vi "CTE_Analysis_Suite_InputMaker.vi"(11 "File Save Path":path=path "C:/TestInputMaker") -> ()   [LabVIEW 2012]
panel:
  in  "Crystal Symmetry":string(combo)="Monoclinic"
  out "Ready":bool=TRUE
  in  "New Phase":bool
  in  "Submit":bool
  in  "stop":bool
  in  "Clear All Fields":bool
  out "Saved As:":string="-25.csv"
  out "Submitted?":bool
  in  "hkl's and d-spacings (Å)":refnum<k7>(container) caption="hkl's and d-spacings (A)"
  in  "Error gamma":dbl
  in  "Error beta":dbl
  in  "Error alpha":dbl
  in  "Error c":dbl
  in  "Error b":dbl
  in  "Error a":dbl
  in  "Temp (°C)":dbl=25.0
  in  "gamma":dbl
  in  "beta":dbl
  in  "alpha":dbl
  in  "c":dbl
  in  "b":dbl
  in  "a":dbl
  in  "Chemical Formula or File Name (no subscripts)":string="FileName1"
  in  "Phase Name":string="NewPhase1"
  # "CTEAS InputMaker v0.2"
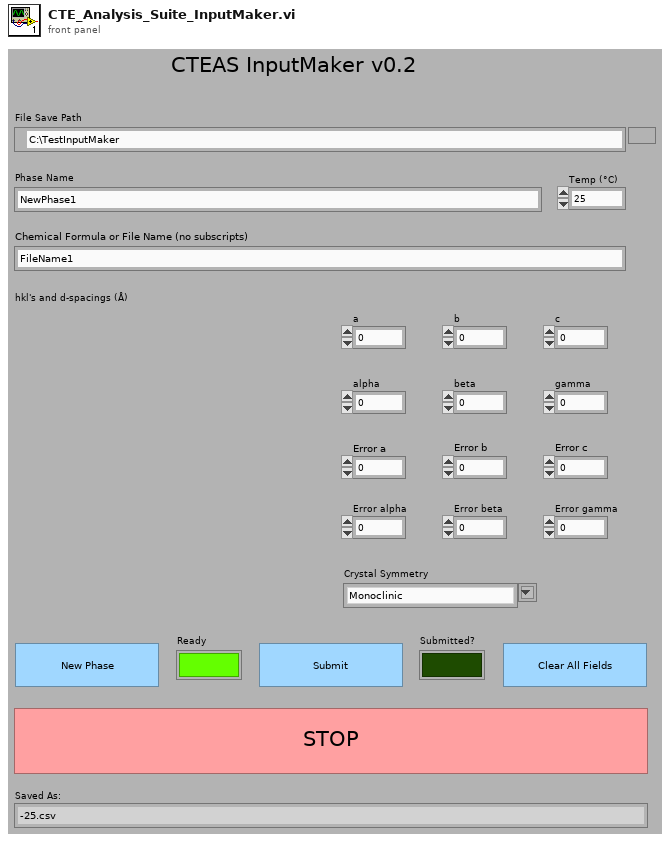
[diagram p1: front panel]
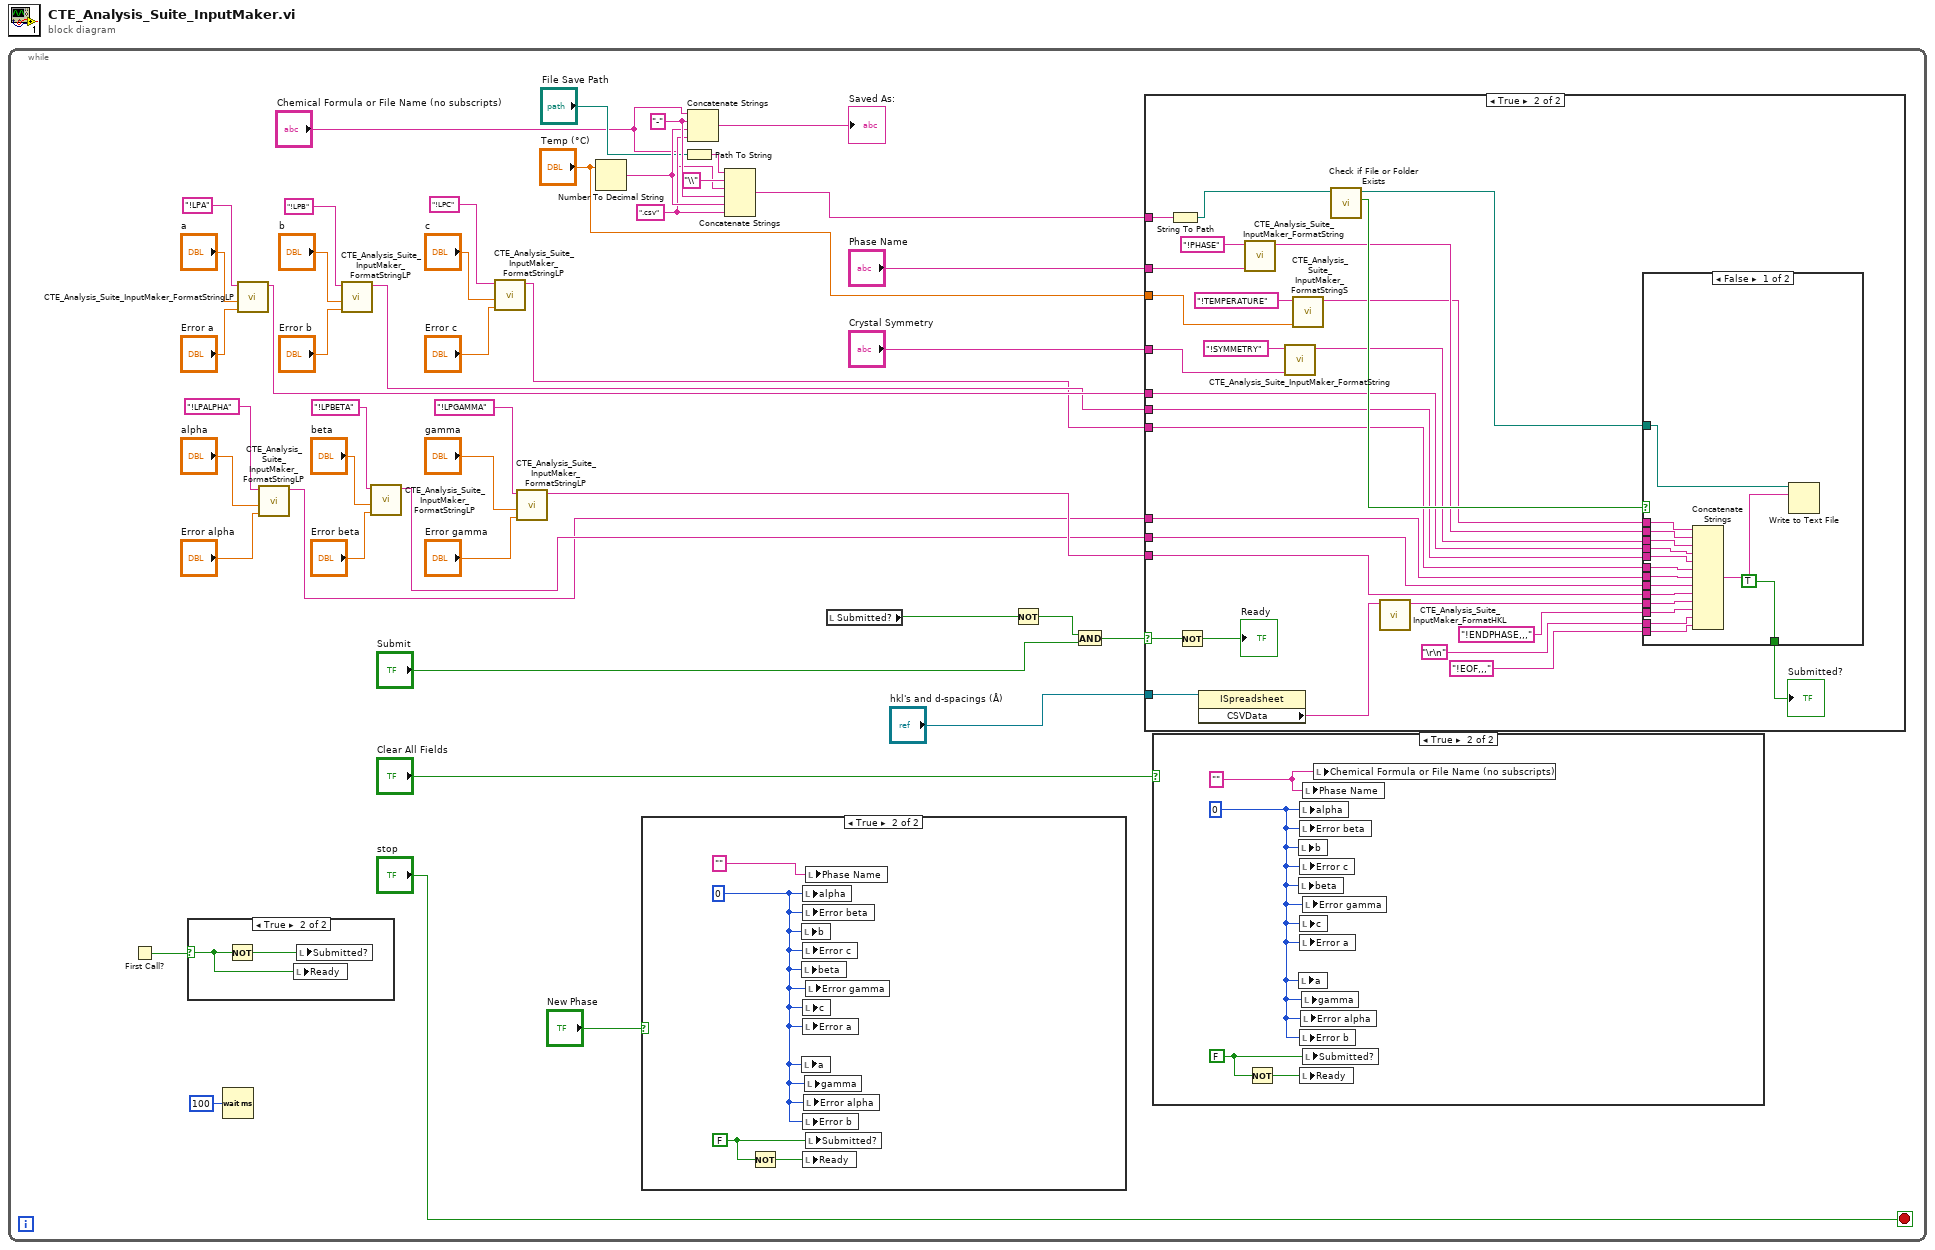
[diagram p0: block diagram]
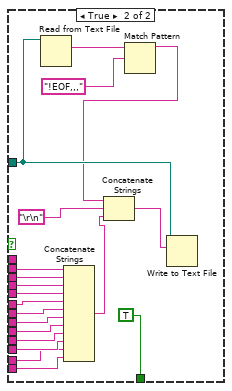
[diagram p6: hidden frame]
diagram:
  n1 = while {
    stop <- "stop" stop-if-true
    w41 = ".csv" ("string")
    w43 = "-" ("string")
    n2 = First Call?() -> (First Call?: T/F=w30:bool)
    n3 = case shown="True" w30 {
      selector: w30 -> [_ w51]
      frame False {
      }
      frame True {
        n4 = Not(x=w51) -> (.not. x?=w52:bool)
        n5 = local write "Ready"(w51) -> ()
        n6 = local write "Submitted?"(w52) -> ()
      }
    }
    n7 = Wait (ms)(milliseconds to wait=u32 100) -> ()  [unwired: 1 out]
    n8 = call "CTE_Analysis_Suite_InputMaker_FormatStringLP.vi"("ERROR"="Error a", "VALUE"="a", "NAME"="!LPA") -> ("Output"=w9:string)  [unwired: 8 in]
    n9 = call "CTE_Analysis_Suite_InputMaker_FormatStringLP.vi"("ERROR"="Error alpha", "VALUE"="alpha", "NAME"="!LPALPHA") -> ("Output"=w4:string)  [unwired: 8 in]
    n10 = call "CTE_Analysis_Suite_InputMaker_FormatStringLP.vi"("ERROR"="Error b", "VALUE"="b", "NAME"="!LPB") -> ("Output"=w8:string)  [unwired: 8 in]
    n11 = call "CTE_Analysis_Suite_InputMaker_FormatStringLP.vi"("ERROR"="Error beta", "VALUE"="beta", "NAME"="!LPBETA") -> ("Output"=w5:string)  [unwired: 8 in]
    n12 = call "CTE_Analysis_Suite_InputMaker_FormatStringLP.vi"("ERROR"="Error c", "VALUE"="c", "NAME"="!LPC") -> ("Output"=w7:string)  [unwired: 8 in]
    n13 = call "CTE_Analysis_Suite_InputMaker_FormatStringLP.vi"("ERROR"="Error gamma", "VALUE"="gamma", "NAME"="!LPGAMMA") -> ("Output"=w6:string)  [unwired: 8 in]
    n14 = Number To Decimal String(number="Temp (°C)") -> (decimal integer string=w42:string)  [unwired: 1 in]
    n15 = case shown="True" "New Phase" {
      frame False {
      }
      frame True {
        w50 = FALSE
        w48 = 0
        n16 = Not(x=w50) -> (.not. x?=w49:bool)
        n17 = local write "b"(w48) -> ()
        n18 = local write "beta"(w48) -> ()
        n19 = local write "a"(w48) -> ()
        n20 = local write "alpha"(w48) -> ()
        n21 = local write "Error beta"(w48) -> ()
        n22 = local write "Error c"(w48) -> ()
        n23 = local write "c"(w48) -> ()
        n24 = local write "Error a"(w48) -> ()
        n25 = local write "Error b"(w48) -> ()
        n26 = local write "Ready"(w49) -> ()
        n27 = local write "Error alpha"(w48) -> ()
        n28 = local write "gamma"(w48) -> ()
        n29 = local write "Phase Name"("") -> ()
        n30 = local write "Error gamma"(w48) -> ()
        n31 = local write "Submitted?"(w50) -> ()
      }
    }
    n32 = Path To String(path="File Save Path") -> (string=w44:string)
    n33 = Concatenate Strings("Chemical Formula or File Name (no subscripts)", w43, w42, w41) -> (→"Saved As:":string)
    n34 = Concatenate Strings(w44, "\\" ("string"), "Chemical Formula or File Name (no subscripts)", w43, w42, w41) -> (w39:string)
    n35 = local read "Submitted?"() -> (w31:bool)
    n36 = Not(x=w31) -> (.not. x?=w32:bool)
    n37 = And(x=w32, y="Submit") -> (x .and. y?=w34:bool)
    n38 = case shown="True" w34 {
      selector: w34 -> [_ w77]
      tunnel: "hkl's and d-spacings (Å)" -> [_ w84]
      tunnel: w39 -> [_ w83]
      tunnel: "Phase Name" -> [_ w75]
      tunnel: "Temp (°C)" -> [_ w74]
      tunnel: "Crystal Symmetry" -> [_ w71]
      tunnel: w9 -> [_ w59]
      tunnel: w8 -> [_ w60]
      tunnel: w7 -> [_ w64]
      tunnel: w6 -> [_ w67]
      tunnel: w5 -> [_ w66]
      tunnel: w4 -> [_ w65]
      frame False {
      }
      frame True {
        n39 = String To Path(string=w83) -> (path=w82:path)
        n40 = Not(x=w77) -> (.not. x?=→"Ready":bool)
        n41 = property class="ISpreadsheet"(reference=w84) -> ("CSVData"=w70:string)  [unwired: 1 in, 2 out]
        n42 = call "CTE_Analysis_Suite_InputMaker_FormatString.vi"("VALUE"=w75, "NAME"="!PHASE") -> ("Output"=w62:string)  [unwired: 9 in]
        n43 = call "CTE_Analysis_Suite_InputMaker_FormatString.vi"("VALUE"=w71, "NAME"="!SYMMETRY") -> ("Output"=w63:string)  [unwired: 9 in]
        n44 = call "CTE_Analysis_Suite_InputMaker_FormatStringS.vi"("VALUE"=w74, "NAME"="!TEMPERATURE") -> ("Output"=w61:string)  [unwired: 9 in]
        n45 = call <vilib>:"Check if File or Folder Exists.vi"("path"=w82) -> ("file or folder exists?"=w81:bool, "dup path"=w80:path)  [unwired: 8 in, 1 out]
        n46 = call "CTE_Analysis_Suite_InputMaker_FormatHKL.vi"("HKLs and D-Spacings"=w70) -> ("Output"=w68:string)  [unwired: 10 in]
        n47 = case shown="False" w81 {
          tunnel: w80 -> [w100 w118]
          tunnel: [TRUE TRUE] -> w79
          tunnel: "!ENDPHASE,,," -> [w98 w116]
          tunnel: w68 -> [w97 w115]
          tunnel: w67 -> [w96 w114]
          tunnel: w66 -> [w95 w113]
          tunnel: w65 -> [w94 w112]
          tunnel: w64 -> [w93 w111]
          tunnel: w63 -> [w92 w110]
          tunnel: w62 -> [w91 w109]
          tunnel: w61 -> [w90 _]
          tunnel: w60 -> [w88 w107]
          tunnel: w59 -> [w87 w106]
          tunnel: "!EOF,,," -> [w85 w104]
          tunnel: "\r\n" -> [w86 w105]
          frame False {
            n48 = Concatenate Strings(w90, w91, w92, w87, w88, w93, w94, w95, w96, w97, w98, w86, w85) -> (w89:string)
            n49 = Write to Text File(file (use dialog)=w100, text=w89) -> ()  [unwired: 2 in, 3 out]
          }
          frame True {
            n50 = Read from Text File(file (use dialog)=w118) -> (text=w103:string)  [unwired: 3 in, 3 out]
            n51 = Concatenate Strings(w109, w110, w106, w107, w111, w112, w113, w114, w115, w116, w105, w104) -> (w108:string)
            n52 = Match Pattern(string=w103, regular expression="!EOF,,,") -> (before substring=w101:string)  [unwired: 1 in, 3 out]
            n53 = Concatenate Strings(w101, "\r\n", w108) -> (w119:string)
            n54 = Write to Text File(file (use dialog)=w118, text=w119) -> ()  [unwired: 2 in, 3 out]
          }
        }
        "Submitted?" <- w79
      }
    }
    n55 = case shown="True" "Clear All Fields" {
      frame False {
      }
      frame True {
        w53 = FALSE
        w56 = ""
        w55 = 0
        n56 = Not(x=w53) -> (.not. x?=w54:bool)
        n57 = local write "b"(w55) -> ()
        n58 = local write "beta"(w55) -> ()
        n59 = local write "a"(w55) -> ()
        n60 = local write "alpha"(w55) -> ()
        n61 = local write "Error beta"(w55) -> ()
        n62 = local write "Error c"(w55) -> ()
        n63 = local write "c"(w55) -> ()
        n64 = local write "Error a"(w55) -> ()
        n65 = local write "Error b"(w55) -> ()
        n66 = local write "Ready"(w54) -> ()
        n67 = local write "Error alpha"(w55) -> ()
        n68 = local write "gamma"(w55) -> ()
        n69 = local write "Phase Name"(w56) -> ()
        n70 = local write "Error gamma"(w55) -> ()
        n71 = local write "Submitted?"(w53) -> ()
        n72 = local write "Chemical Formula or File Name (no subscripts)"(w56) -> ()
      }
    }
  }
